vi "Ic_AxiconLens.vi"(8 "error in (no error)":errorcluster, 9 "Pixel Pitch 0:20um_or_ 1:12.5um":u8, 10 "Top level / πrad.":dbl, 11 "2D array in (LCOS size buf)":u8[][](array[numeric])) -> (0 "error out":errorcluster, 3 "2D array out":u8[][](array[numeric]))   [LabVIEW 2016]
uses:
  LabVIEW2018/Image_Control.dll
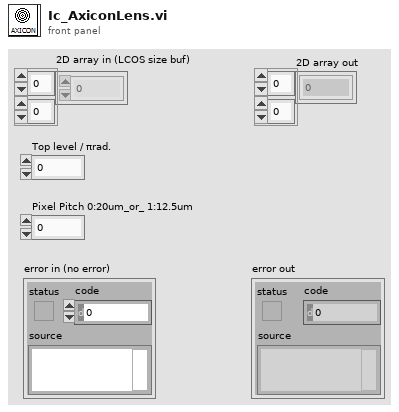
[diagram p1: front panel]
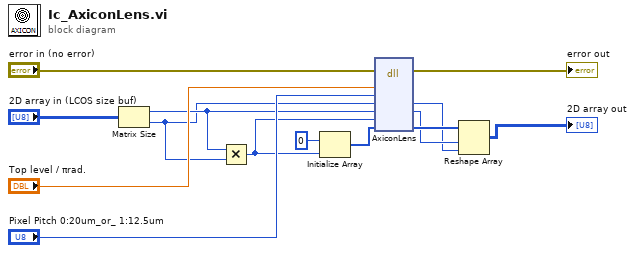
[diagram p0: block diagram]
diagram:
  n1 = Matrix Size(0:"2D array in (LCOS size buf)") -> (1:w9:i32, 2:w8:i32)
  n2 = Multiply(x=w9, y=w8) -> (x*y=w6:i32)
  n3 = Initialize Array(u8 0 ("要素"), w6) -> (w5:u8[])
  n4 = dll-call lib="C:/Users/hs5921/Desktop/LabVIEW2018/Image_Control.dll" fn="AxiconLens"(error in="error in (no error)", "TopLevelRad"="Top level / πrad.", "PixelPitch0_20um_or_1_1.25um"="Pixel Pitch 0:20um_or_ 1:12.5um", "X_pixel_target"=w8, "Y_pixel_target"=w9, "targetDataSize"=w6, "1DArrayOut"=w5) -> (error out=→"error out":errorcluster, "X_pixel_target"=w2:i32, "Y_pixel_target"=w3:i32, "1DArrayOut"=w4:u8[])  [unwired: 6 in, 1 out]
  n5 = Reshape Array(w4, w3, w2) -> (→"2D array out":u8[][])
